vi "Find all vis in current project.vi"(4 "error in":errorcluster, 7 "ExcludeDependencies?":bool) -> (0 "error out":errorcluster, 2 "Project name":string, 3 "All VIs in .proj":string[](array[string]))   [LabVIEW 2010]
doc: "This .vi returns references to all the .vi's under the My Computer section of the current project This requires that only one project is open. \n\nIf multiple projects are open, he current project has to have the conditional disable symbol : ProjectName with the project name present, and the subdiagram filled out in the subvi."
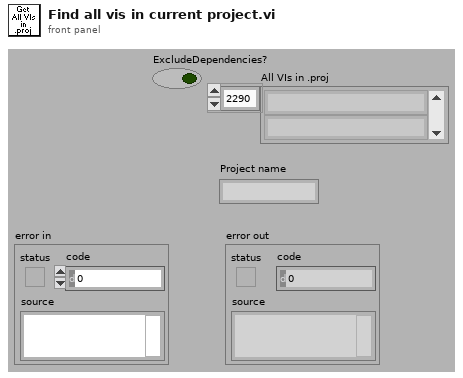
[diagram p1: front panel]
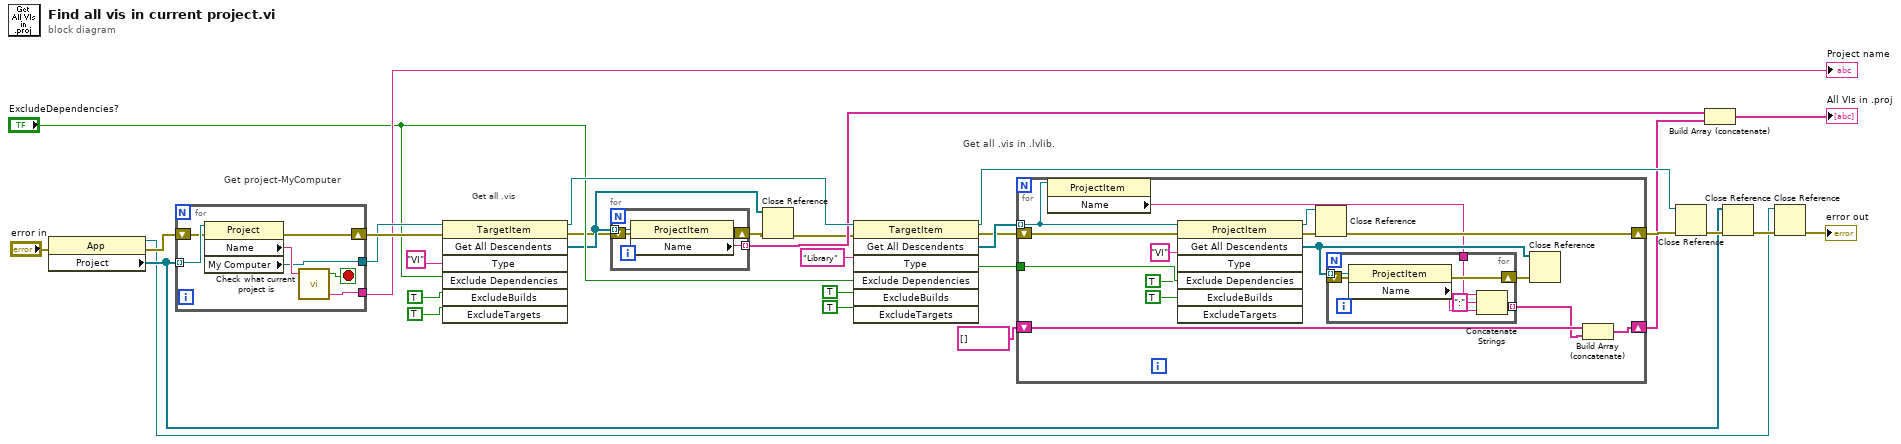
[diagram p0: block diagram]
diagram:
  # "Get project-MyComputer"
  # "Get all .vis in .lvlib."
  # "Get all .vis"
  n1 = property class="App"(error in="error in") -> (reference out=w19:refnum<vi>, error out=w26:errorcluster, "Project"=w21:refnum<vi>[])  [unwired: 1 in]
  n2 = for {
    tunnel: w21 -> [w36] mode=indexing
    shift-right: [w33] -> w29
    shift-left: w26 -> [w34]
    tunnel: [w32] -> w27
    tunnel: [w31] -> w28
    stop <- w37 stop-if-true
    n3 = property class="Project"(reference=w36, error in=w34) -> (error out=w33:errorcluster, "Name"=w35:string, "My Computer"=w31:refnum<vi>)  [unwired: 1 out]
    n4 = call "Check what current project is.vi"("Project Name"=w35) -> ("Project"=w32:string, "Input = Current Project,\nor project not defined?"=w37:bool)  [unwired: 3 out]
  }
  "Project name" <- w27
  n5 = invoke class="TargetItem" method="Get All Descendents"(reference=w28, error in=w29, "Type"="VI", "Exclude Dependencies"="ExcludeDependencies?", "ExcludeBuilds"=TRUE, "ExcludeTargets"=TRUE ("ExcludeBuilds")) -> (reference out=w17:refnum<vi>, error out=w3:errorcluster, "All Descendents"=w4:refnum<vi>[])  [unwired: 1 in, 4 out]
  n6 = for {
    tunnel: w4 -> [w41] mode=indexing
    tunnel: [w40] -> w6 mode=indexing
    shift-right: [w39] -> w5
    shift-left: w3 -> [w38]
    n7 = property class="ProjectItem"(reference=w41, error in=w38) -> (error out=w39:errorcluster, "Name"=w40:string)  [unwired: 1 out]
  }
  n8 = Close Reference(reference=w4, error in (no error)=w5) -> (error out=w2:errorcluster)
  n9 = invoke class="TargetItem" method="Get All Descendents"(reference=w17, error in=w2, "Type"="Library", "Exclude Dependencies"="ExcludeDependencies?", "ExcludeBuilds"=TRUE, "ExcludeTargets"=TRUE) -> (reference out=w16:refnum<vi>, error out=w10:errorcluster, "All Descendents"=w12:refnum<vi>[])  [unwired: 1 in, 4 out]
  n10 = for {
    tunnel: w12 -> [w43] mode=indexing
    tunnel: "ExcludeDependencies?" -> [w55]
    shift-right: [w49] -> w9
    shift-left: w10 -> [w50]
    shift-right: [w47] -> w1
    shift-left: string[] [] -> [w48]
    n11 = property class="ProjectItem"(reference=w43) -> ("Name"=w42:string)  [unwired: 1 in, 2 out]
    n12 = invoke class="ProjectItem" method="Get All Descendents"(reference=w43, error in=w50, "Type"="VI", "Exclude Dependencies"=w55, "ExcludeBuilds"=TRUE, "ExcludeTargets"=TRUE) -> (reference out=w51:refnum<vi>, error out=w52:errorcluster, "All Descendents"=w46:refnum<vi>[])  [unwired: 1 in, 4 out]
    n13 = Close Reference(reference=w51, error in (no error)=w52) -> (error out=w49:errorcluster)
    n14 = for {
      tunnel: w46 -> [w63] mode=indexing
      shift-right: [w62] -> w45
      shift-left: _ -> [w61]
      tunnel: [w59] -> w44 mode=indexing
      tunnel: w42 -> [w58]
      n15 = property class="ProjectItem"(reference=w63, error in=w61) -> (error out=w62:errorcluster, "Name"=w60:string)  [unwired: 1 out]
      n16 = Concatenate Strings(w58, ":" ("string"), w60) -> (w59:string)
    }
    n17 = Close Reference(reference=w46, error in (no error)=w45) -> ()  [unwired: 1 out]
    n18 = Build Array (concatenate)(w48, w44) -> (w47:string[])
  }
  n19 = Close Reference(reference=w16, error in (no error)=w9) -> (error out=w22:errorcluster)
  n20 = Build Array (concatenate)(w6, w1) -> (→"All VIs in .proj":string[])
  n21 = Close Reference(reference=w21, error in (no error)=w22) -> (error out=w20:errorcluster)
  n22 = Close Reference(reference=w19, error in (no error)=w20) -> (error out=→"error out":errorcluster)
